vi "autogetglobal.vi"() -> ()   [LabVIEW 2011]
panel:
  out "lua_tointeger":i32
  out "lua_gettop":i32
  out "error out":errorcluster
  out "lua_type":i32(ring) items=["LUA_TNONE"=-1, "LUA_TNIL"=0, "LUA_TBOOLEAN"=1, "LUA_TLIGHTUSERDATA"=2, "LUA_TNUMBER "=3, "LUA_TSTRING"=4, "LUA_TTABLE"=5, "LUA_TFUNCTION"=6, "LUA_TUSERDATA"=7, "LUA_TTHREAD"=8, "LUA_NUMTAGS "=9]
  in  "const char *name":string
  in  "lua_State *L":u64
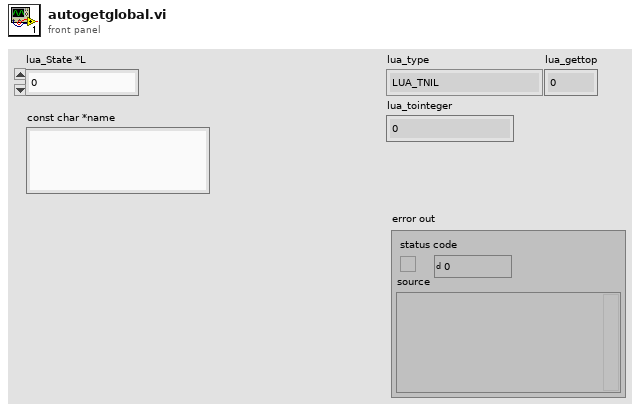
[diagram p1: front panel]
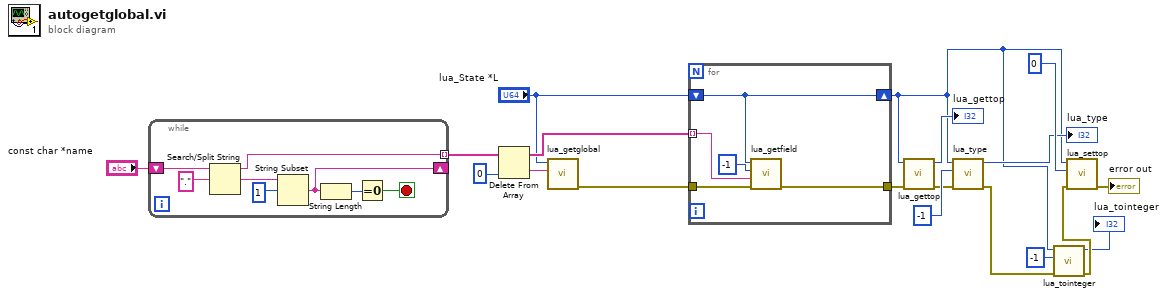
[diagram p0: block diagram]
diagram:
  n1 = while {
    shift-right: [w23] -> _
    shift-left: "const char *name" -> [w26]
    tunnel: [w20] -> w18 mode=indexing
    stop <- w21 stop-if-true
    n2 = Search/Split String(string=w26, search string/char (-)="." ("正则表达式")) -> (substring before match=w20:string, match + rest of string=w25:string)  [unwired: 1 in, 1 out]
    n3 = String Subset(string=w25, offset (0)=1 ("偏移量(0)")) -> (substring=w23:string)  [unwired: 1 in]
    n4 = String Length(string=w23) -> (length=w22:i32)
    n5 = Equal To 0?(x=w22) -> (x = 0?=w21:bool)
  }
  n6 = Delete From Array(array=w18, index=0 ("索引")) -> (deleted portion=w16:string, array with subset deleted=w15:string[])  [unwired: 1 in]
  n7 = call "lua_getglobal.vi"("const char *name"=w16, "lua_State *L"="lua_State *L") -> ("error out"=w11:errorcluster)  [unwired: 9 in]
  n8 = for {
    tunnel: w11 -> [w30]
    tunnel: w15 -> [w32] mode=indexing
    tunnel: [w31] -> w8
    shift-right: [w29] -> w2
    shift-left: "lua_State *L" -> [w29]
    n9 = call "lua_getfield.vi"("error in"=w30, "const char *name"=w32, "int index"=-1, "lua_State *L"=w29) -> ("error out"=w31:errorcluster)  [unwired: 7 in]
  }
  n10 = call "lua_gettop.vi"("error in"=w8, "lua_State *L"=w2) -> ("error out"=w7:errorcluster, "lua_gettop"=→"lua_gettop":i32)  [unwired: 8 in]
  n11 = call "lua_type.vi"("error in"=w7, "int index"=-1, "lua_State *L"=w2) -> ("error out"=w5:errorcluster, "lua_type"=→"lua_type":i32)  [unwired: 7 in]
  n12 = call "lua_tointeger.vi"("error in"=w5, "index"=-1, "lua_State *L"=w2) -> ("error out"=w4:errorcluster, "lua_tointeger"=→"lua_tointeger":i32)  [unwired: 7 in]
  n13 = call "lua_settop.vi"("error in"=w4, "index"=0, "lua_State *L"=w2) -> ("error out"=→"error out":errorcluster)  [unwired: 8 in]
